vi "SetWavelength.vi"(8 "error in (no error)":errorcluster, 9 "Interaction Type":string, 10 "Wavelength, nm":dbl, 11 "Topas In":refnum<k24>) -> (0 "error out":errorcluster, 2 "IsSuccess":bool, 3 "Topas out":refnum<k24>)   [LabVIEW 2017]
uses:
  D:/upwork/Laser Measurement Tool/Topas4PublicAPI/NET_SDK/Topas4Lib.dll
  Topas4PublicAPI/NET_SDK/Topas4Lib.dll
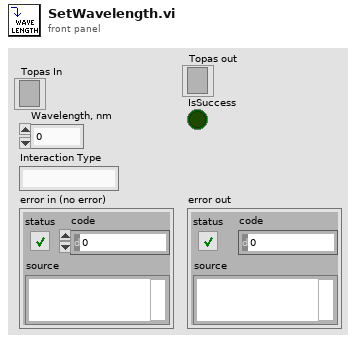
[diagram p1: front panel]
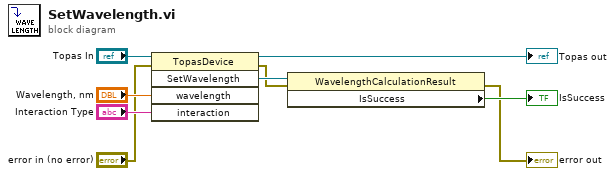
[diagram p0: block diagram]
diagram:
  n1 = invoke class="TopasDevice" method="SetWavelength"(reference="Topas In", error in="error in (no error)", "wavelength"="Wavelength, nm", "interaction"="Interaction Type") -> (reference out=→"Topas out":refnum<k24>, error out=w4:errorcluster, "SetWavelength"=w5:refnum<k24>)  [unwired: 1 in, 2 out]
  n2 = property class="WavelengthCalculationResult"(reference=w5, error in=w4) -> (error out=→"error out":errorcluster, "IsSuccess"=→"IsSuccess":bool)  [unwired: 1 out]
